vi "Camera Test 2.vi"() -> ()   [LabVIEW 2016, in "Test2.lvrbt"]
uses:
  Test2.lvrbt
  <vilib>/NXT/Block Support/NXT_InputPort.ctl
  <vilib>/NXT/Hardware/Plugins/Tetrix DC Motor/TetrixDCMotorAddress.ctl
  <vilib>/NXT/LegoClasses/BrickReference/BrickReference.lvclass
  <vilib>/NXT/Subs/LVHSConnector.ctl
  <vilib>/NXT/NXTIO Xnodes/NXTIONodeSubVIs/TETRIX IO Move DC Motors.vi
  <vilib>/NXT/NXTIO Xnodes/NXTIOXNode/NXTIO.xnode
  <vilib>/NXT/NXTIO Xnodes/AddressXNode/NXTIOAddress.xnode
  <vilib>/NXT/NXTIO Xnodes/NXTIONodeSubVIs/TETRIX IO Stop DC Motors.vi
  <vilib>/NXT/Dual Mode Library/Waits/Wait_Num.vi
  <vilib>/NXT/Hardware/Plugins/Tetrix 180 deg Servo/Tetrix180ServoAddress.ctl
  <vilib>/NXT/NXTIO Xnodes/NXTIONodeSubVIs/TETRIX IO Move Servos.vi
  <vilib>/NXT/Dual Mode Library/Waits/Wait_EV3_Color_Color.vi
  <vilib>/NXT/Subs/ColorSensorColors.ctl
panel:
  out "Power":bool
  out "X Upper Left":u8
  out "X Lower Right":u8
  out "Y Lower Right":u8
  out "Y Upper Left":u8
  out "Count":u8
  out "Color":u8
  in  "Cluster":T1 {"Tracking Mode" items=["Disable Tracking", "Get First Object", "Get n th Object", "Enable Tracking", "Sort Objects  by size", "Sort Objects  by Colors", "Illumination on ", "Illumination Off", "Write Colormap", "Read Colormap", "Line tracking mode", "Object Tracking mode"]}
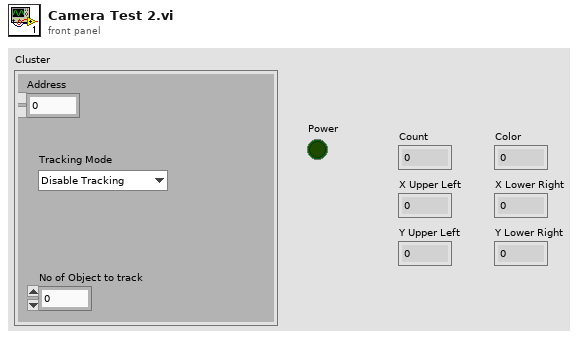
[diagram p1: front panel]
types:
  T1 = cluster{"Address":dbl, "No of Object to track":dbl, "Tracking Mode":u8}
  T2 = typedef "NXT_InputPort.ctl" = u32
  T3 = typedef "ColorSensorColors.ctl" = enum16{"No Color", "Black", "Blue", "Green", "Yellow", "Red", "White", "Brown"}
  T4 = cluster{"Tracking Mode":u8, "Object Number to Track":u8, "Address":u8}
  T5 = typedef "Tetrix180ServoAddress.ctl" = i32
  T6 = cluster{"Tetrix180Servo":T5, "Tetrix180Servo":T5, "Tetrix180Servo":T5, "Tetrix180Servo":T5, "Tetrix180Servo":T5, "Tetrix180Servo":T5}
  T7 = typedef "LVHSConnector.ctl" = refnum<class "BrickReference.lvclass">
  T8 = typedef "TetrixDCMotorAddress.ctl" = i32
  T9 = cluster{"TetrixDCMotor":T8, "TetrixDCMotor 2":T8}
  T10 = cluster{"Total Tracked Objects":u8, "Color":u8, "X Upper Left":u8, "Y Upper Left":u8, "X Lower Right":u8, "Y Lower Right":u8, "Status (boolean)":bool}
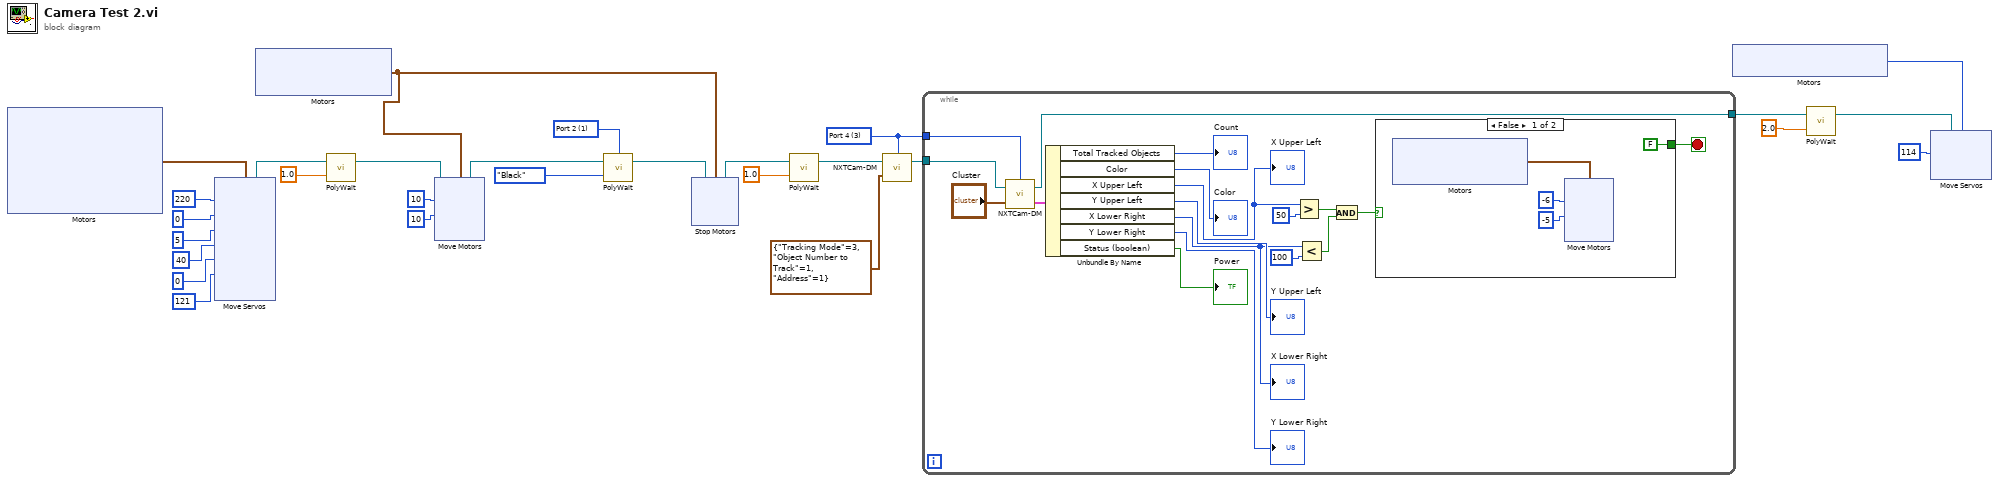
[diagram p0: block diagram]
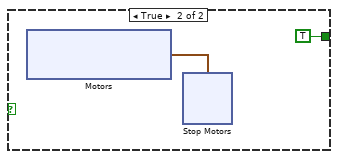
[diagram p2: hidden frame]
diagram:
  w1 = T2 1 items=["Port 1", "Port 2", "Port 3", "Port 4"] ("Port (Port 1)")
  w26 = T2 3 items=["Port 1", "Port 2", "Port 3", "Port 4"] ("Input Port")
  n1 = xnode "Motors"() -> ("Motor"=w14:T6)
  n2 = xnode "Move Servos"("Position 6"=u8 121, "Position 5"=u8 0, "Position 4"=u8 40, "Position 3"=u8 5, "Position 2"=u8 0, "Position 1"=u8 220, "Motors"=w14) -> ("NXT/EV3"=w6:T7)  [unwired: 1 in]
  n3 = xnode "Motors"() -> ("Motor"=w23:cluster{"TetrixDCMotor":T8, "TetrixDCMotor":T8})
  n4 = call-poly <vilib>:"PolyWait.vi"("Time (1 sec)"=sgl 1.0, "NXT/EV3"=w6) -> ("NXT/EV3"=w2:T7)  [unwired: 2 in]
  n5 = xnode "Move Motors"("Power/Speed 2"=i8 10, "Power/Speed 1"=i8 10, "Motors"=w23, "NXT/EV3"=w2) -> ("NXT/EV3"=w4:T7)
  n6 = call-poly <vilib>:"PolyWait.vi"("Color (Red)"=ColorSensorColors."Black", "NXT/EV3"=w4, "Port (Port 1)"=w1) -> ("NXT/EV3"=w3:T7)  [unwired: 1 in]
  n7 = xnode "Stop Motors"("Motors"=w23, "NXT/EV3"=w3) -> ("NXT/EV3"=w22:T7)
  n8 = call-poly <vilib>:"PolyWait.vi"("Time (1 sec)"=sgl 1.0, "NXT/EV3"=w22) -> ("NXT/EV3"=w21:T7)  [unwired: 2 in]
  n9 = call "NXTCam-DM.vi"("Input of NXTCam"=T4 {"Tracking Mode"=3, "Object Number to Track"=1, "Address"=1}, "NXT"=w21, "Input Port"=w26) -> ("NXT dup"=w28:T7)  [unwired: 1 out]
  n10 = while {
    tunnel: w26 -> [w44]
    tunnel: w28 -> [w43]
    tunnel: [w29] -> w18
    stop <- w30 stop-if-true
    n11 = call "NXTCam-DM.vi"("Input of NXTCam"="Cluster", "NXT"=w43, "Input Port"=w44) -> ("Output of NXTCam"=w39:T10, "NXT dup"=w29:T7)
    n12 = Unbundle By Name(w39) -> ("Total Tracked Objects"=→"Count":u8, "Color"=→"Color":u8, "X Upper Left"=w37:u8, "Y Upper Left"=→"Y Upper Left":u8, "X Lower Right"=w35:u8, "Y Lower Right"=→"Y Lower Right":u8, "Status (boolean)"=→"Power":bool)
    "X Upper Left" <- w37
    "X Lower Right" <- w35
    n13 = Greater?(x=w37, y=u8 50) -> (0:w33:bool)
    n14 = Less?(x=w35, y=u8 100) -> (x < y?=w32:bool)
    n15 = And(x=w33, y=w32) -> (x .and. y?=w31:bool)
    n16 = case shown="False" w31 {
      tunnel: [FALSE TRUE] -> w30
      frame False {
        n17 = xnode "Motors"() -> ("Motor"=w50:cluster{"TetrixDCMotor":T8, "TetrixDCMotor":T8})
        n18 = xnode "Move Motors"("Power/Speed 2"=i8 -5, "Power/Speed 1"=i8 -6, "Motors"=w50) -> ()  [unwired: 1 in, 1 out]
      }
      frame True {
        n19 = xnode "Motors"() -> ("Motor"=w61:cluster{"TetrixDCMotor":T8, "TetrixDCMotor":T8})
        n20 = xnode "Stop Motors"("Motors"=w61) -> ()  [unwired: 1 in, 1 out]
      }
    }
  }
  n21 = xnode "Motors"() -> ("Motor"=w15:T5)
  n22 = call-poly <vilib>:"PolyWait.vi"("Time (1 sec)"=sgl 2.0, "NXT/EV3"=w18) -> ("NXT/EV3"=w17:T7)  [unwired: 2 in]
  n23 = xnode "Move Servos"("Position 1"=u8 114, "Motors"=w15, "NXT/EV3"=w17) -> ()  [unwired: 1 out]
